vi "SocketHandle_0 - 複製.vi"(7 "Mode":enum16{"Open", "Read", "Write", "Close"}(ring), 8 "error in (no error)":errorcluster, 9 "data in":string, 10 "Port":u16=6342, 11 "Machine":string="localhost") -> (0 "error out":errorcluster, 3 "data out":string)   [LabVIEW 2011]
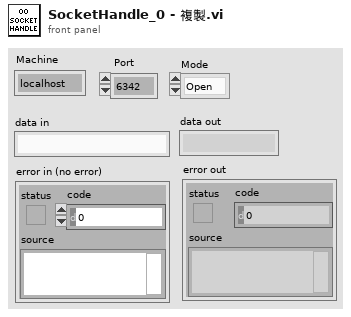
[diagram p1: front panel]
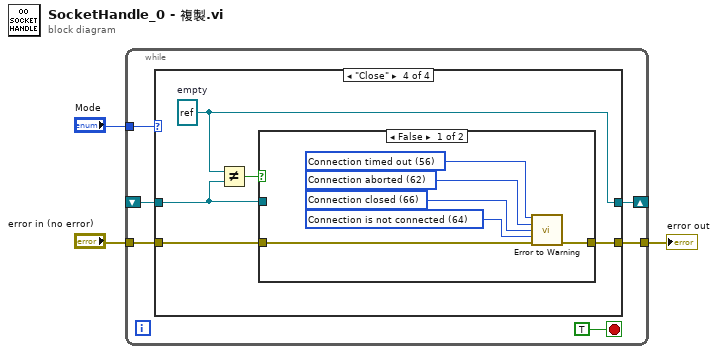
[diagram p0: block diagram]
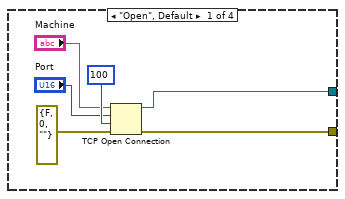
[diagram p2: hidden frame]
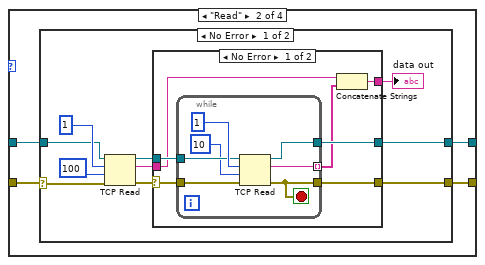
[diagram p3: hidden frame]
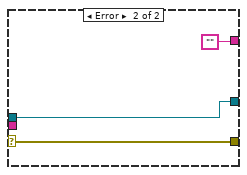
[diagram p4: hidden frame]
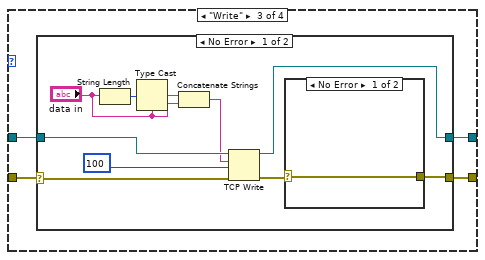
[diagram p6: hidden frame]
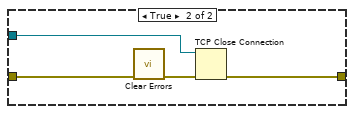
[diagram p9: hidden frame]
diagram:
  n1 = while {
    shift-right: [w9] -> _
    shift-left: _ -> [w6]
    tunnel: "Mode" -> [w5]
    tunnel: "error in (no error)" -> [w7]
    tunnel: [w8] -> w1
    stop <- TRUE stop-if-true
    n2 = case shown="\"Close\"" w5 {
      tunnel: [w14 w19 w51 w68] -> w9
      tunnel: [w12 w16 w50 w71] -> w8
      tunnel: w7 -> [_ w17 w49 w70]
      tunnel: w6 -> [_ w18 w52 w67]
      frame "Open", Default {
        n3 = TCP Open Connection(address="Machine", remote port or service name="Port", timeout ms (60000)=100, error in (no error)=errorcluster {"status"=FALSE, "code"=0, "source"=""} ("error constant")) -> (connection ID=w14:refnum<k5>, error out=w12:errorcluster)  [unwired: 1 out]
      }
      frame "Read" {
        n4 = case shown="No Error" w17 {
          selector: w17 -> [w20 w47]
          tunnel: [w24 w47] -> w16
          tunnel: [w23 w48] -> w19
          tunnel: w18 -> [w22 w48]
          frame No Error {
            n5 = TCP Read(connection ID=w22, bytes to read=1, error in (no error)=w20, 9:100 ("timeout ms (25000)")) -> (connection ID out=w28:refnum<k5>, data out=w29:string, error out=w26:errorcluster)  [unwired: 1 in]
            n6 = case shown="No Error" w26 {
              selector: w26 -> [w36 w45]
              tunnel: w29 -> [w31 _]
              tunnel: w28 -> [w35 w46]
              tunnel: [w34 w46] -> w23
              tunnel: [w33 ""] -> w21
              tunnel: [w30 w45] -> w24
              frame No Error {
                n7 = while {
                  tunnel: w36 -> [w43]
                  tunnel: w35 -> [w41]
                  tunnel: [w40] -> w34
                  tunnel: [w39] -> w32 mode=indexing
                  tunnel: [w38] -> w30
                  stop <- w38 stop-if-true
                  n8 = TCP Read(connection ID=w41, bytes to read=1, error in (no error)=w43, 9:10 ("timeout ms (25000)")) -> (connection ID out=w40:refnum<k5>, data out=w39:string, error out=w38:errorcluster)  [unwired: 1 in]
                }
                n9 = Concatenate Strings(w31, w32) -> (w33:string)
              }
              frame Error {
              }
            }
            "data out" <- w21
          }
          frame Error {
          }
        }
      }
      frame "Write" {
        n10 = case shown="No Error" w49 {
          selector: w49 -> [w60 w65]
          tunnel: w52 -> [w62 w66]
          tunnel: [w57 w66] -> w51
          tunnel: [w58 w65] -> w50
          frame No Error {
            n11 = String Length(string="data in") -> (length=w56:i32)
            n12 = Type Cast(type="data in", x=w56) -> (*(type *) &x=w55:string)
            n13 = Concatenate Strings(w55, "data in") -> (w53:string)
            n14 = TCP Write(connection ID=w62, data in=w53, error in (no error)=w60, 9:100 ("timeout ms (25000)")) -> (connection ID out=w57:refnum<k5>, error out=w59:errorcluster)  [unwired: 1 out]
            n15 = case shown="No Error" w59 {
              selector: w59 -> [w63 w64]
              tunnel: [w63 w64] -> w58
              frame No Error {
              }
              frame Error {
              }
            }
          }
          frame Error {
          }
        }
      }
      frame "Close" {
        w68 = refnum<k5> refnum  # empty
        n16 = Not Equal?(x=w68, y=w67) -> (x != y?=w69:bool)
        n17 = case shown="False" w69 {
          tunnel: [w76 w81] -> w71
          tunnel: w70 -> [w77 w80]
          tunnel: w67 -> [_ w78]
          frame False {
            w72 = 64 items=["No Error", "Argument Error", "Memory Full", "Out of Zone", "End of File", "File Already Open", "Generic File IO Error", "File Not Found", "File Permission Error", "Disk Full", "Duplicate Path", "Too Many Files Open", "Not Enabled", "Resource File Not Found", "Cannot Add Resource", "Resource Not Found", "Image Not Found", "Image Memory Error", "Pen Does Not Exist", "Config Bad Type", "Config Token Not Found", "Config Parse Error", "Config Memory Error", "Bad External Code Format", "Bad External Code Offset", "External Code Not Present", "Null Window", "Destroy Window Mixup", "Null Menu", "Print Aborted", "Bad Print Record", "Print Driver Error", "Windows Error During Print", "Memory Error During Print", "Print Dialog Error", "Generic Print Error", "Invalid Device Refnum", "Device Not Found", "Device Parameter Error", "Device Unit Error", "Can't Open Device", "Device Call Aborted", "Generic Error", "Cancelled By User", "Object ID Too Low", "Object ID Too High", "Object Not In Heap", "Unknown Heap", "Bad DefProc ID", "DefProc Not In Table", "Message Out Of Range", "Null Method", "Unknown Message", "Manager Call Not Supported", "Bad address", "Connection In progress", "Connection timed out", "Connection is already in progress", "Network attribute not supported", "Network error", "Address in use", "System out of memory", "Connection aborted", "Connection refused", "Connection is not connected", "Connection is already connected", "Connection closed", "Initialize error (interapplication manager)", "Bad occurrence", "Wait on unbound occurrence handler", "Occurrence queue overflow", "Bad path", "Semaphore not signaled", "Unrecognized type (interapplication manager)"] ("1st Error to Convert")
            w73 = 66 items=["No Error", "Argument Error", "Memory Full", "Out of Zone", "End of File", "File Already Open", "Generic File IO Error", "File Not Found", "File Permission Error", "Disk Full", "Duplicate Path", "Too Many Files Open", "Not Enabled", "Resource File Not Found", "Cannot Add Resource", "Resource Not Found", "Image Not Found", "Image Memory Error", "Pen Does Not Exist", "Config Bad Type", "Config Token Not Found", "Config Parse Error", "Config Memory Error", "Bad External Code Format", "Bad External Code Offset", "External Code Not Present", "Null Window", "Destroy Window Mixup", "Null Menu", "Print Aborted", "Bad Print Record", "Print Driver Error", "Windows Error During Print", "Memory Error During Print", "Print Dialog Error", "Generic Print Error", "Invalid Device Refnum", "Device Not Found", "Device Parameter Error", "Device Unit Error", "Can't Open Device", "Device Call Aborted", "Generic Error", "Cancelled By User", "Object ID Too Low", "Object ID Too High", "Object Not In Heap", "Unknown Heap", "Bad DefProc ID", "DefProc Not In Table", "Message Out Of Range", "Null Method", "Unknown Message", "Manager Call Not Supported", "Bad address", "Connection In progress", "Connection timed out", "Connection is already in progress", "Network attribute not supported", "Network error", "Address in use", "System out of memory", "Connection aborted", "Connection refused", "Connection is not connected", "Connection is already connected", "Connection closed", "Initialize error (interapplication manager)", "Bad occurrence", "Wait on unbound occurrence handler", "Occurrence queue overflow", "Bad path", "Semaphore not signaled", "Unrecognized type (interapplication manager)"] ("1st Error to Convert")
            w74 = 62 items=["No Error", "Argument Error", "Memory Full", "Out of Zone", "End of File", "File Already Open", "Generic File IO Error", "File Not Found", "File Permission Error", "Disk Full", "Duplicate Path", "Too Many Files Open", "Not Enabled", "Resource File Not Found", "Cannot Add Resource", "Resource Not Found", "Image Not Found", "Image Memory Error", "Pen Does Not Exist", "Config Bad Type", "Config Token Not Found", "Config Parse Error", "Config Memory Error", "Bad External Code Format", "Bad External Code Offset", "External Code Not Present", "Null Window", "Destroy Window Mixup", "Null Menu", "Print Aborted", "Bad Print Record", "Print Driver Error", "Windows Error During Print", "Memory Error During Print", "Print Dialog Error", "Generic Print Error", "Invalid Device Refnum", "Device Not Found", "Device Parameter Error", "Device Unit Error", "Can't Open Device", "Device Call Aborted", "Generic Error", "Cancelled By User", "Object ID Too Low", "Object ID Too High", "Object Not In Heap", "Unknown Heap", "Bad DefProc ID", "DefProc Not In Table", "Message Out Of Range", "Null Method", "Unknown Message", "Manager Call Not Supported", "Bad address", "Connection In progress", "Connection timed out", "Connection is already in progress", "Network attribute not supported", "Network error", "Address in use", "System out of memory", "Connection aborted", "Connection refused", "Connection is not connected", "Connection is already connected", "Connection closed", "Initialize error (interapplication manager)", "Bad occurrence", "Wait on unbound occurrence handler", "Occurrence queue overflow", "Bad path", "Semaphore not signaled", "Unrecognized type (interapplication manager)"] ("1st Error to Convert")
            w75 = 56 items=["No Error", "Argument Error", "Memory Full", "Out of Zone", "End of File", "File Already Open", "Generic File IO Error", "File Not Found", "File Permission Error", "Disk Full", "Duplicate Path", "Too Many Files Open", "Not Enabled", "Resource File Not Found", "Cannot Add Resource", "Resource Not Found", "Image Not Found", "Image Memory Error", "Pen Does Not Exist", "Config Bad Type", "Config Token Not Found", "Config Parse Error", "Config Memory Error", "Bad External Code Format", "Bad External Code Offset", "External Code Not Present", "Null Window", "Destroy Window Mixup", "Null Menu", "Print Aborted", "Bad Print Record", "Print Driver Error", "Windows Error During Print", "Memory Error During Print", "Print Dialog Error", "Generic Print Error", "Invalid Device Refnum", "Device Not Found", "Device Parameter Error", "Device Unit Error", "Can't Open Device", "Device Call Aborted", "Generic Error", "Cancelled By User", "Object ID Too Low", "Object ID Too High", "Object Not In Heap", "Unknown Heap", "Bad DefProc ID", "DefProc Not In Table", "Message Out Of Range", "Null Method", "Unknown Message", "Manager Call Not Supported", "Bad address", "Connection In progress", "Connection timed out", "Connection is already in progress", "Network attribute not supported", "Network error", "Address in use", "System out of memory", "Connection aborted", "Connection refused", "Connection is not connected", "Connection is already connected", "Connection closed", "Initialize error (interapplication manager)", "Bad occurrence", "Wait on unbound occurrence handler", "Occurrence queue overflow", "Bad path", "Semaphore not signaled", "Unrecognized type (interapplication manager)"] ("1st Error to Convert")
            n18 = call <vilib>:"Error to Warning.vi"("1st Error to Convert"=w75, "2nd Error to Convert"=w74, "3rd Error to Convert"=w73, "4th Error to Convert"=w72, "error in"=w77) -> ("warning out"=w76:errorcluster)  [unwired: 10 in]
          }
          frame True {
            n19 = call <vilib>:"Clear Errors.vi"("error in (no error)"=w80) -> ("error out"=w79:errorcluster)  [unwired: 6 in]
            n20 = TCP Close Connection(connection ID=w78, error in (no error)=w79) -> (error out=w81:errorcluster)  [unwired: 2 out]
          }
        }
      }
    }
  }
  "error out" <- w1
